vi "普通cable读写操作 vice.vi"(10 "Channel":u8 max=5 step=1, 11 "VISA":refnum<visa-resource-name>="COM6") -> (2 "result":bool)   [LabVIEW 2011]
panel:
  out "message":string
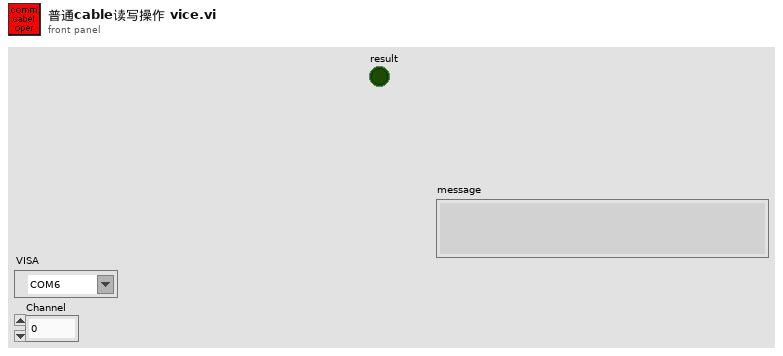
[diagram p1: front panel]
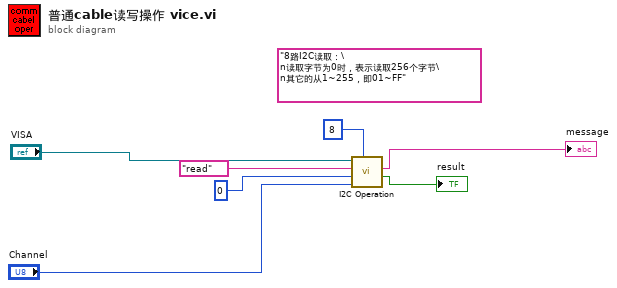
[diagram p0: block diagram]
diagram:
  (unwired) "8路I2C读取：\n读取字节为0时，表示读取256个字节\n其它的从1~255，即01~FF"
  n1 = call "I2C Operation.vi"("size"=8, "Channel"="Channel", "address"=u8 0, "mode"="read", "VISA"="VISA") -> ("result"=→"result":bool, "message"=→"message":string)  [unwired: 3 in, 2 out]
